vi "Cross Power Spectrum.vi"(3 "dt":dbl=1.0 format="%0.2f", 4 "Signal Y (V)":dbl[](array[numeric]), 5 "Signal X (V)":dbl[](array[numeric])) -> (0 "df":dbl format="%0.2f", 1 "Cross Power XY Spectrum Phase (radians)":dbl[](array[numeric]), 2 "Cross Power XY Spectrum Mag (V^2rms)":dbl[](array[numeric]))   [LabVIEW 2010, in "NI_AALPro.lvlib"]
doc: "Computes the single-sided, scaled, cross power spectrum of two real-time signals."
uses:
  NI_AALPro.lvlib
  Cross Power (DBL).vi
panel:
  # "Cross Power Spectrum"
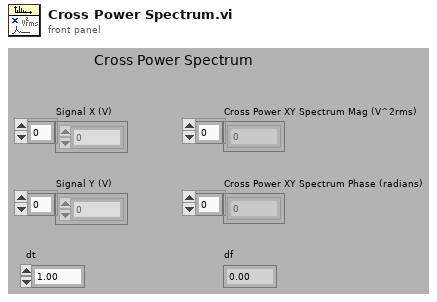
[diagram p1: front panel]
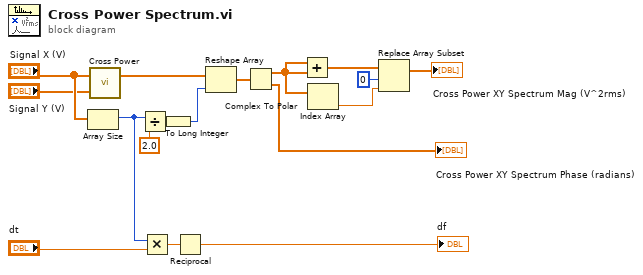
[diagram p0: block diagram]
diagram:
  n1 = Array Size(array="Signal X (V)") -> (size(s)=w13:i32)
  n2 = call-poly "Cross Power.vi"("Y"="Signal Y (V)", "X"="Signal X (V)") -> ("Sxy"=w9:cdb[])  [unwired: 1 out]
  n3 = Divide(x=w13, y=2.0) -> (x/y=w10:dbl)
  n4 = Multiply(x=w13, y="dt") -> (x*y=w16:dbl)
  n5 = To Long Integer(number=w10) -> (32bit integer=w7:i32)
  n6 = Reciprocal(x=w16) -> (1/x=→"df":dbl)
  n7 = Reshape Array(w9, w7) -> (w8:cdb[])
  n8 = Complex To Polar(r * e^(i*theta)=w8) -> (r=w5:dbl[], theta=→"Cross Power XY Spectrum Phase (radians)":dbl[])
  n9 = Add(x=w5, y=w5) -> (x+y=w4:dbl[])
  n10 = Index Array(array=w5) -> (element=w3:dbl)  [unwired: 1 in]
  n11 = Replace Array Subset(array=w4, new element=w3, index=0) -> (→"Cross Power XY Spectrum Mag (V^2rms)":dbl[])
